vi "stop.vi"(8 "error in (no error)":errorcluster, 9 "InternalCommandId.lvclass":refnum<class "InternalCommandId.lvclass">, 10 "ElectrometerController int":refnum<class "ElectrometerController.lvclass">, 11 "ReadingState in":refnum<class "ManualReadingState.lvclass">) -> (0 "error out":errorcluster, 2 "ElectrometerController out":refnum<class "ElectrometerController.lvclass">, 3 "ReadingState out":refnum<class "ManualReadingState.lvclass">)   [LabVIEW 2016, in "ManualReadingState.lvclass"]
uses:
  ManualReadingState.lvclass
  ElectrometerController/ElectrometerController.lvclass
  InternalCommandId/InternalCommandId.lvclass
  ts_electrometeruserevents/Typedefs/StateValue.ctl
  ts_electrometeruserevents/Typedefs/MeasuringPeriod.ctl
  ElectrometerController/ElectrometerController.lvclass/ElectrometerController.ctl
  ElectrometerController/readBuffer.vi
  ElectrometerState.lvclass
  ts_electrometeruserevents/Typedefs/ElectrometerTypedefs.lvlib
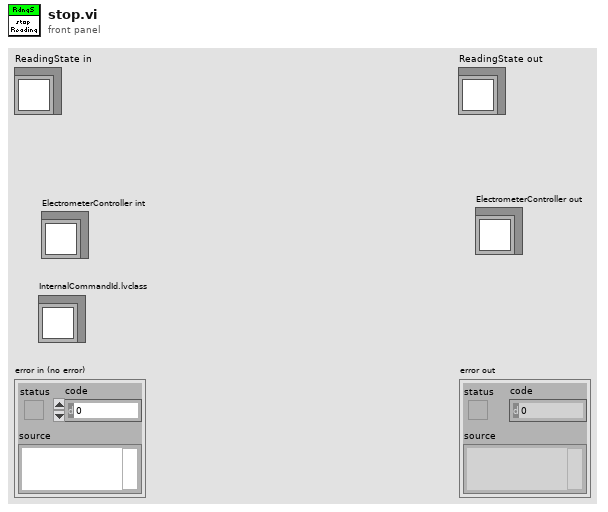
[diagram p1: front panel]
types:
  T1 = typedef "ElectrometerTypedefs.lvlib/MeasuringPeriod.ctl" = enum16{"Initial", "End"}
  T2 = typedef "ElectrometerTypedefs.lvlib/StateValue.ctl" = enum16{"", "DisabledState", "EnabledState", "FaultState", "OffState", "StandbyState", "ReadyState", "ConfiguringState", "ManualReadingState", "UntilIntensityReadingState", "SetDurationReadingState", "BufferReadingState"}
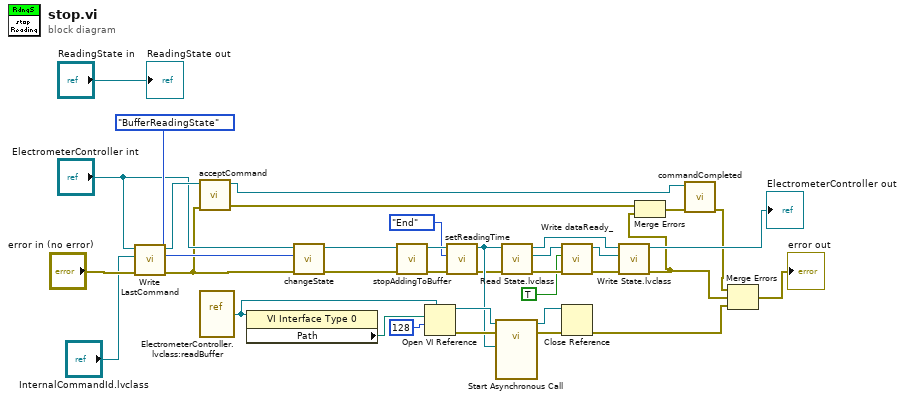
[diagram p0: block diagram]
diagram:
  n1 = call "Write LastCommand.vi"("error in (no error)"="error in (no error)", "InternalCommandId.lvclass"="InternalCommandId.lvclass", "ElectrometerController in"="ElectrometerController int") -> ("error out"=w1:errorcluster, "ElectrometerController out"=w8:refnum<class "ElectrometerController.lvclass">)  [unwired: 7 in]
  n2 = call "acceptCommand.vi"("error in (no error)"=w1, "ElectrometerController in"=w8) -> ("error out"=w6:errorcluster, "ElectrometerController out"=w5:refnum<class "ElectrometerController.lvclass">)  [unwired: 8 in]
  n3 = vi-ref "ElectrometerController.lvclass:readBuffer.vi"() -> (w19:refnum<vi>)
  n4 = property class="VI Interface Type 0"(reference=w19) -> ("Path"=w23:path)  [unwired: 1 in, 2 out]
  n5 = call "changeState.vi"("error in (no error)"=w1, "StateValue"=StateValue."BufferReadingState", "ElectrometerController in"="ElectrometerController int") -> ("error out"=w26:errorcluster, "ElectrometerController out"=w27:refnum<class "ElectrometerController.lvclass">)  [unwired: 7 in]
  n6 = call "stopAddingToBuffer.vi"("error in (no error)"=w26, "ElectrometerController in"=w27) -> ("error out"=w14:errorcluster, "ElectrometerController out"=w17:refnum<class "ElectrometerController.lvclass">)  [unwired: 8 in]
  n7 = Open VI Reference(type specifier VI Refnum (for type only)=w19, vi path=w23, options=128) -> (vi reference=w21:refnum<vi>, error out=w20:errorcluster)  [unwired: 3 in]
  n8 = call "setReadingTime.vi"("error in (no error)"=w14, "Period"=MeasuringPeriod."End", "ElectrometerController in"=w17) -> ("error out"=w15:errorcluster, "ElectrometerController out"=w16:refnum<class "ElectrometerController.lvclass">)  [unwired: 7 in]
  n9 = call-by-ref "Start Asynchronous Call"(reference=w21, error in=w20, "ElectrometerController in"=w16) -> (reference out=w24:refnum<vi>, error out=w25:errorcluster)  [unwired: 9 in, 2 out]
  n10 = call-dynamic "Read State.lvclass.vi"("error in (no error)"=w15, "ElectrometerController in"=w16) -> ("error out"=w33:errorcluster, "ElectrometerState"=w34:refnum<class "ElectrometerState.lvclass">, "ElectrometerController out"=w30:refnum<class "ElectrometerController.lvclass">)  [unwired: 7 in]
  n11 = call-dynamic "Write dataReady_.vi"("error in (no error)"=w33, "dataReady?"=TRUE, "State in"=w34) -> ("error out"=w29:errorcluster, "State out"=w31:refnum<class "ElectrometerState.lvclass">)  [unwired: 7 in]
  n12 = Close Reference(reference=w24, error in (no error)=w25) -> (error out=w12:errorcluster)
  n13 = call-dynamic "Write State.lvclass.vi"("error in (no error)"=w29, "ElectrometerState"=w31, "ElectrometerController in"=w30) -> ("error out"=w7:errorcluster, "ElectrometerController out"=→"ElectrometerController out":refnum<class "ElectrometerController.lvclass">)  [unwired: 7 in]
  n14 = Merge Errors(w6, w7) -> (w4:errorcluster)
  n15 = call "commandCompleted.vi"("error in (no error)"=w4, "ElectrometerController in"=w5) -> ("error out"=w3:errorcluster)  [unwired: 8 in, 1 out]
  n16 = Merge Errors(w3, w7, w12) -> (→"error out":errorcluster)
  "ReadingState out" <- "ReadingState in"
